vi "Microwave Amplifier Control Panel (No Objects).vi"(8 "error in (no error)":errorcluster) -> (0 "error out":errorcluster)   [LabVIEW 2012]
doc: "(Dynamic) A user-level application that simulates the physical front panel of the Instrument. Provide the user with buttons to manually control features of the instrument, and provide indicators of its current state."
uses:
  Microwave Amp/MicrowaveAmplifier.lvlib
panel:
  in  "VISA Resource Name":refnum<visa-resource-name>="GPIB0::12::INSTR"
  in  "Copy actual to set":bool
  in  "Populate fields with member data":bool
  in  "Read Remaining Time Delay":bool
  in  "Read Amplifier Status/Mode":bool
  in  "Standby":bool
  in  "stop":bool
  out "Mode":u16(ring) items=["SLEEP", "WARM-UP", "STANDBY", "OPERATE", "FAULT"]
  in  "Operate":bool
  in  "Read Reverse Power Out (W)":bool
  in  "Read Reverse Power Out (dBm)":bool
  in  "Read Forward Power Out (W)":bool
  in  "Read Forward Power out (dBm)":bool
  in  "Read Gain":bool
  in  "Set Gain":bool
  out "Remaining Heater Delay Time":dbl[unit]
  out "Reverse Power Out (dBm)":dbl
  out "Reverse Power Out (W)":dbl[unit]
  out "Forward Power Out (dBm)":dbl
  out "Forward Power Out (W)":dbl[unit]
  out "Gain (%)":dbl
  in  "GainSet":dbl
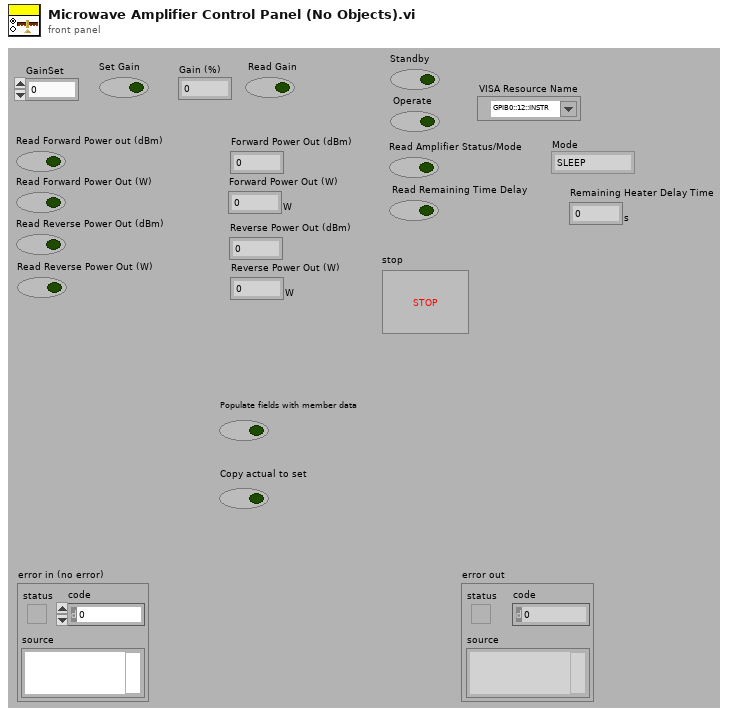
[diagram p1: front panel]
types:
  T1 = cluster{"Gain (%)":dbl, "Forward Power Out (dBm)":dbl, "Forward Power Out (W)":dbl[unit], "Reverse Power Out (dBm)":dbl, "Reverse Power Out (W)":dbl[unit], "Mode":u16, "Remaining Heater Delay Time (s)":dbl[unit]}
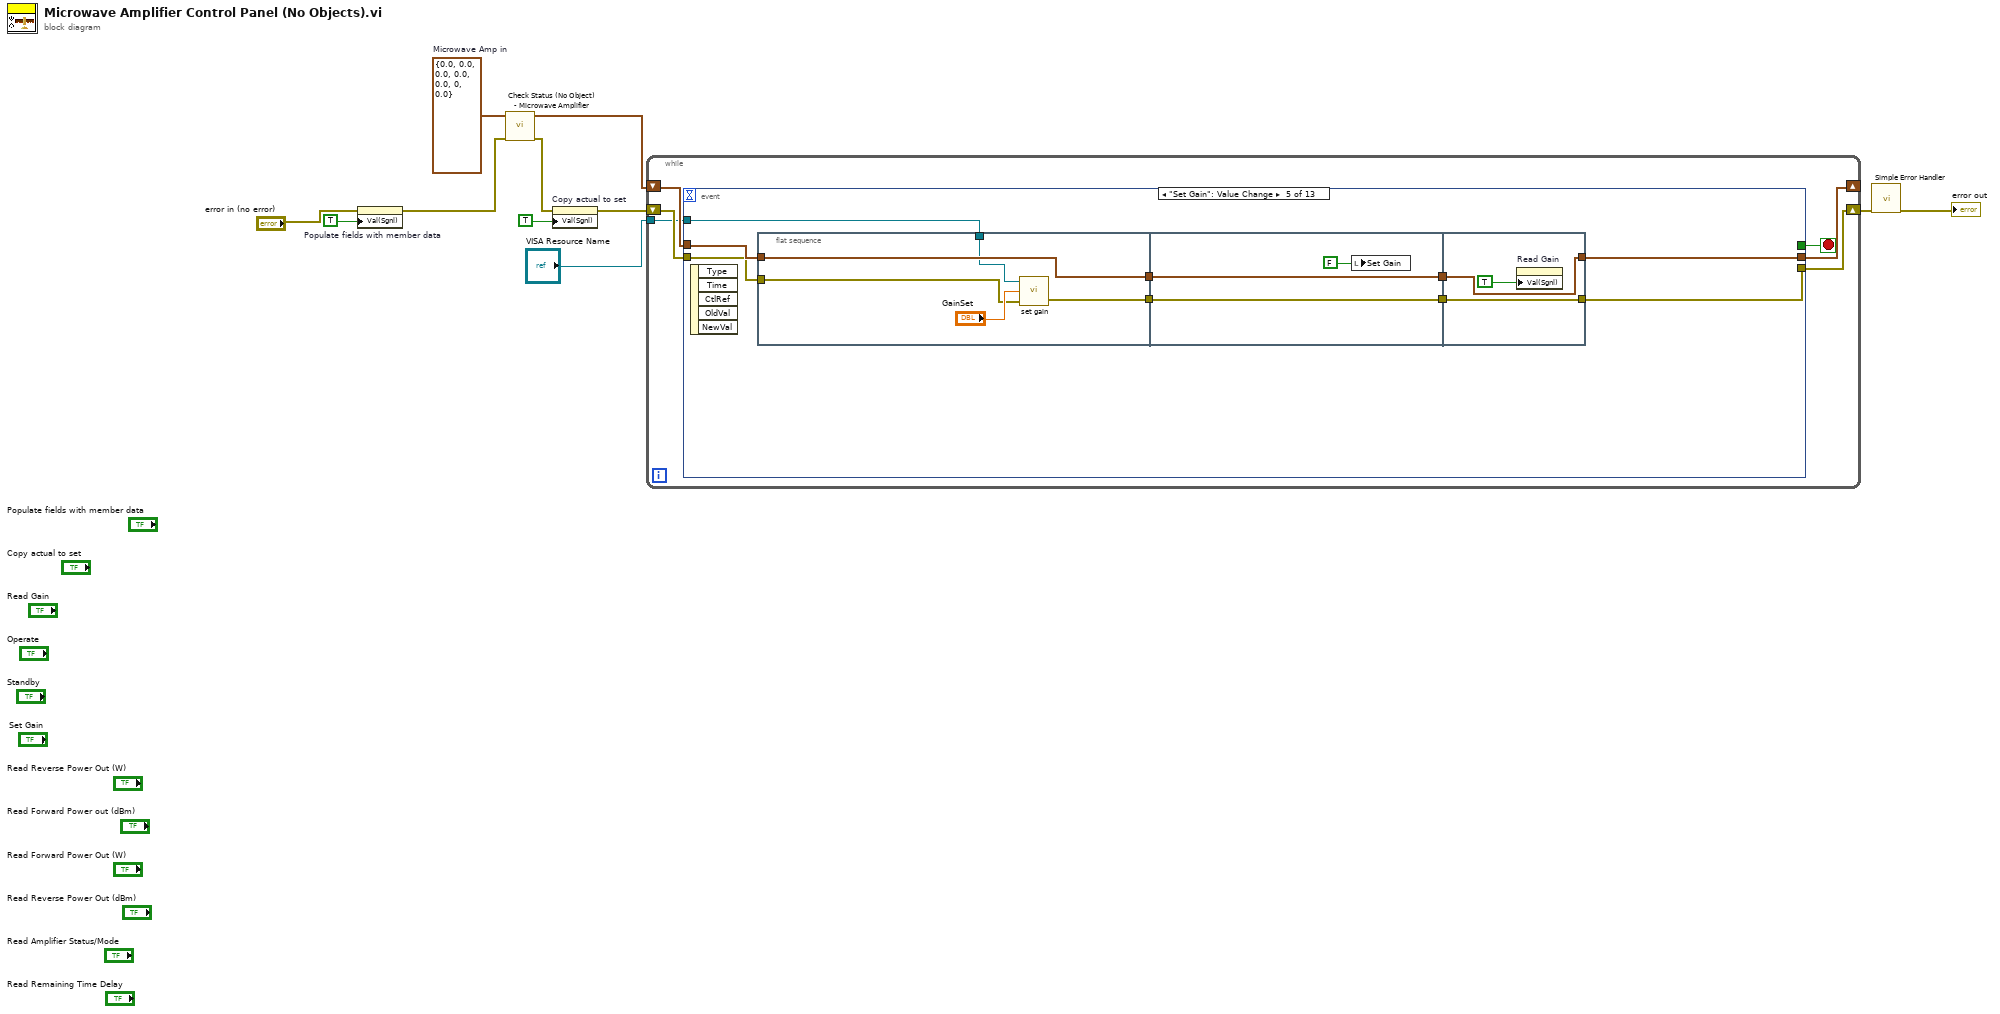
[diagram p0: block diagram]
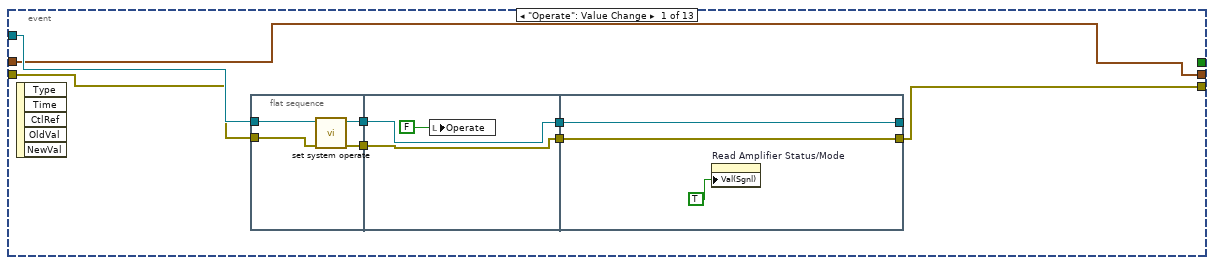
[diagram p2: hidden frame]
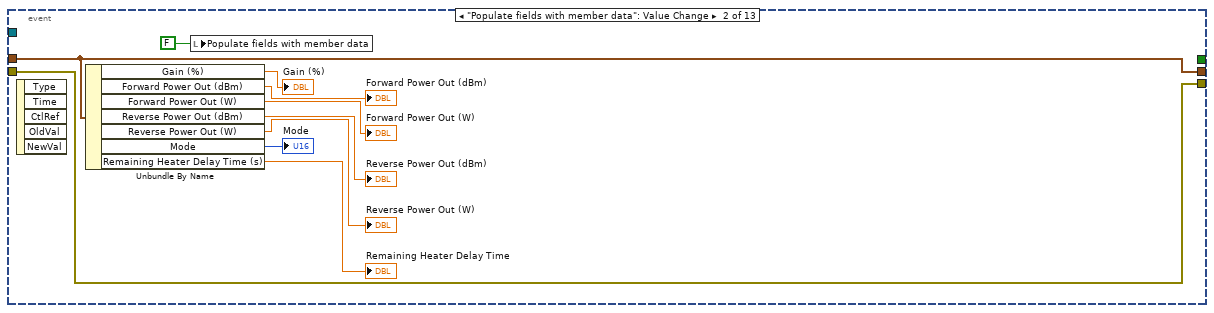
[diagram p3: hidden frame]
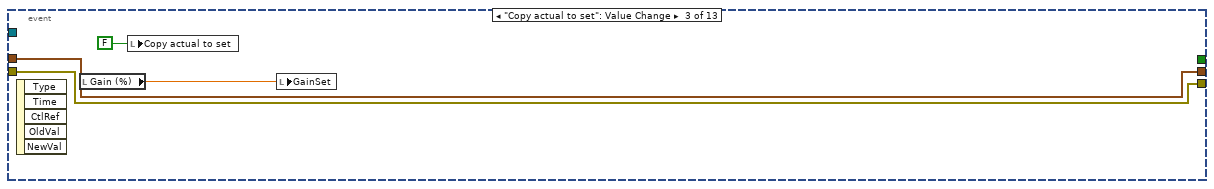
[diagram p4: hidden frame]
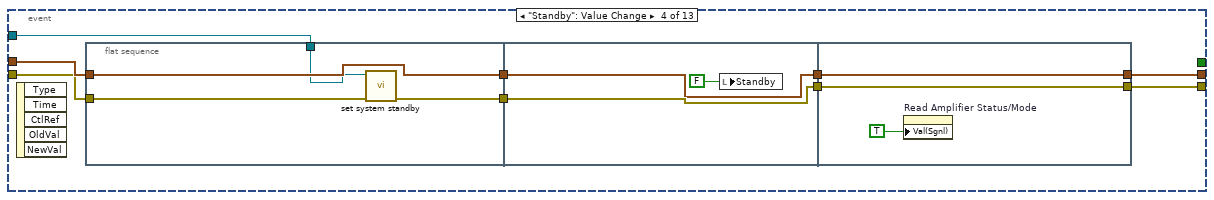
[diagram p5: hidden frame]
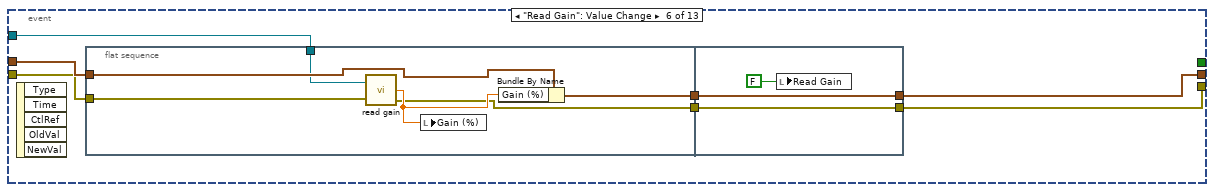
[diagram p6: hidden frame]
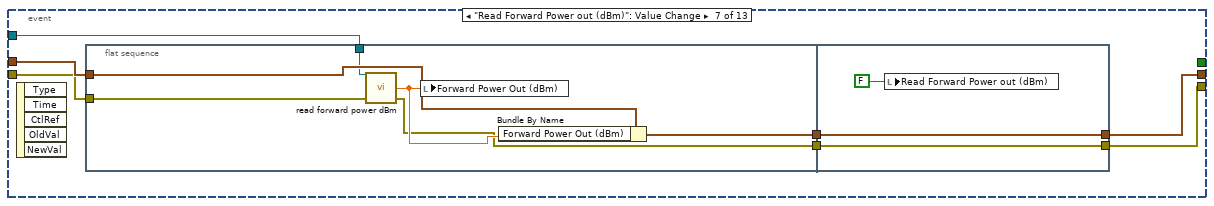
[diagram p7: hidden frame]
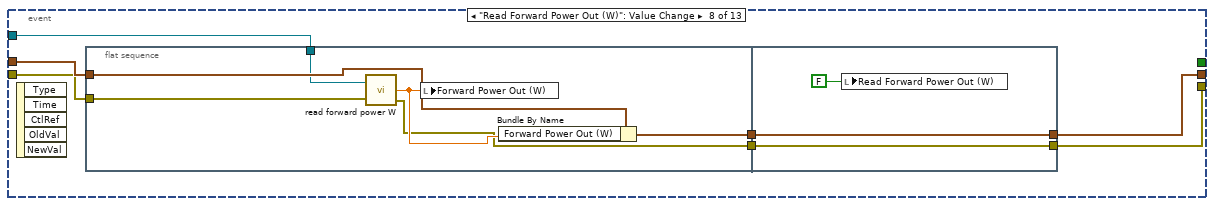
[diagram p8: hidden frame]
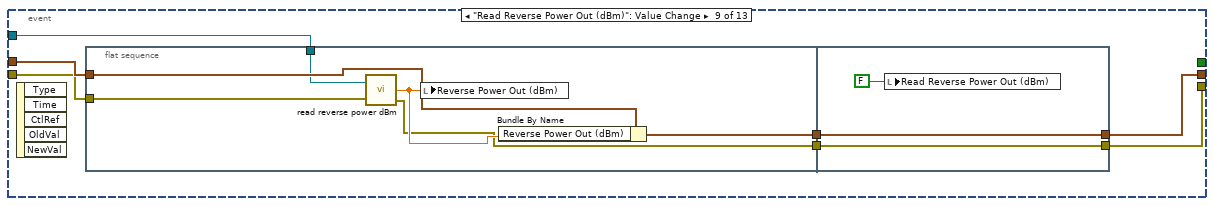
[diagram p9: hidden frame]
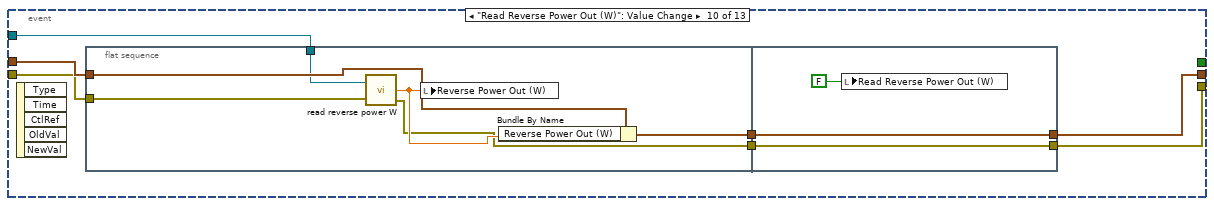
[diagram p10: hidden frame]
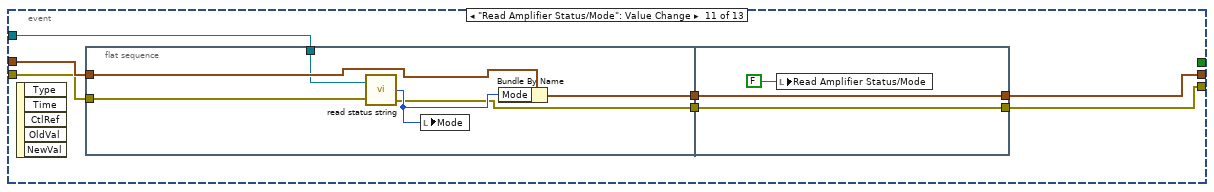
[diagram p11: hidden frame]
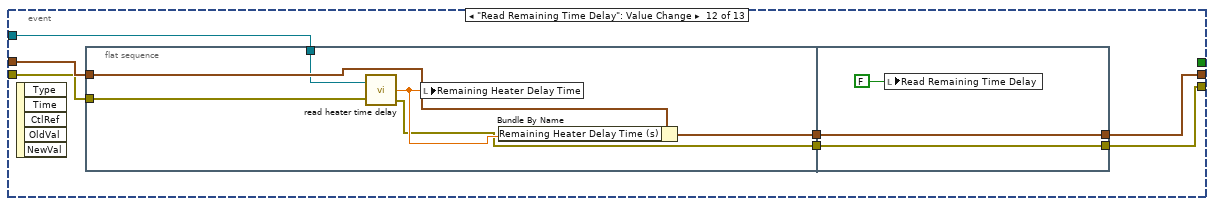
[diagram p12: hidden frame]
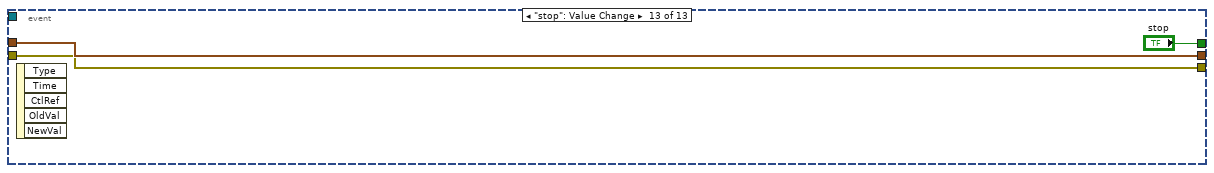
[diagram p13: hidden frame]
diagram:
  w5 = T1 {"Gain (%)"=0.0, "Forward Power Out (dBm)"=0.0, "Forward Power Out (W)"=0.0, "Reverse Power Out (dBm)"=0.0, "Reverse Power Out (W)"=0.0, "Mode"=0, "Remaining Heater Delay Time (s)"=0.0}  # Microwave Amp in
  n1 = property on="Populate fields with member data" class="Bool (strict)"(error in="error in (no error)", "Val(Sgnl)"=TRUE ("Value (Signaling)")) -> (error out=w3:errorcluster)  [unwired: 1 in, 1 out]
  n2 = call "Check Status (No Object) - Microwave Amplifier.vi"("error in (no error)"=w3, "Cluster In"=w5) -> ("error out"=w2:errorcluster, "Cluster Out"=w4:T1)  [unwired: 6 in, 2 out]
  n3 = property on="Copy actual to set" class="Bool (strict)"(error in=w2, "Val(Sgnl)"=TRUE ("Value (Signaling)")) -> (error out=w8:errorcluster)  [unwired: 1 in, 1 out]
  n4 = while {
    shift-right: [w17] -> w11
    shift-left: w8 -> [w14]
    shift-right: [w15] -> _
    shift-left: w4 -> [w13]
    tunnel: "VISA Resource Name" -> [w12]
    stop <- w16 stop-if-true
    n5 = event shown="[4] \"Set Gain\": Value Change" {
      selector: _ -> [_ _ _ _ _ _ _ _ _ _ _ _ _]
      dyn-events: _ -> [_ _ _ _ _ _ _ _ _ _ _ _ _]
      timeout: _ -> [_ _ _ _ _ _ _ _ _ _ _ _ _]
      tunnel: w14 -> [w20 w45 w48 w53 w74 w93 w107 w123 w139 w155 w171 w189 w201]
      tunnel: [w18 w45 w48 w57 w70 w90 w106 w122 w138 w154 w170 w186 w201] -> w17
      tunnel: [_ _ _ _ _ _ _ _ _ _ _ _ "stop"] -> w16
      tunnel: w13 -> [w19 w44 w49 w54 w75 w94 w110 w126 w142 w158 w174 w190 w202]
      tunnel: [w19 w44 w49 w55 w73 w92 w109 w125 w141 w157 w173 w188 w202] -> w15
      tunnel: w12 -> [w21 _ _ w50 w69 w89 w105 w121 w137 w153 w169 w185 _]
      event "Operate": Value Change {
        n6 = event-data() -> ()  [unwired: 1 in, 5 out]
        n7 = flat-sequence {
          tunnel: [w29] -> w25
          tunnel: [w28] -> w24
          tunnel: w20 -> [w27]
          tunnel: w21 -> [w26]
          tunnel: w25 -> [w31]
          tunnel: w24 -> [w30]
          tunnel: [w31] -> w23
          tunnel: [w30] -> w22
          tunnel: [w34] -> w18
          tunnel: [w35] -> _
          tunnel: w23 -> [w35]
          tunnel: w22 -> [w34]
          frame #0 {
            n8 = call "set system operate.vi"("error in (no error)"=w27, "VISA resource name"=w26) -> ("error out"=w28:errorcluster, "VISA resource name out"=w29:refnum<visa-resource-name>)  [unwired: 8 in]
          }
          frame #1 {
            n9 = local write "Operate"(FALSE ("Operate")) -> ()
          }
          frame #2 {
            n10 = property on="Read Amplifier Status/Mode" class="Bool (strict)"("Val(Sgnl)"=TRUE ("Value (Signaling)")) -> ()  [unwired: 2 in, 2 out]
          }
        }
      }
      event "Populate fields with member data": Value Change {
        n11 = event-data() -> ()  [unwired: 1 in, 5 out]
        n12 = Unbundle By Name(w44) -> ("Gain (%)"=→"Gain (%)":dbl, "Forward Power Out (dBm)"=→"Forward Power Out (dBm)":dbl, "Forward Power Out (W)"=→"Forward Power Out (W)":dbl[unit], "Reverse Power Out (dBm)"=→"Reverse Power Out (dBm)":dbl, "Reverse Power Out (W)"=→"Reverse Power Out (W)":dbl[unit], "Mode"=→"Mode":u16, "Remaining Heater Delay Time (s)"=→"Remaining Heater Delay Time":dbl[unit])
        n13 = local write "Populate fields with member data"(FALSE ("Populate fields with member data")) -> ()
      }
      event "Copy actual to set": Value Change {
        n14 = event-data() -> ()  [unwired: 1 in, 5 out]
        n15 = local read "Gain (%)"() -> (w46:dbl)
        n16 = local write "Copy actual to set"(FALSE ("Copy actual to set")) -> ()
        n17 = local write "GainSet"(w46) -> ()
      }
      event "Standby": Value Change {
        n18 = event-data() -> ()  [unwired: 1 in, 5 out]
        n19 = flat-sequence {
          tunnel: [w62] -> w58
          tunnel: [w61] -> w56
          tunnel: w54 -> [w61]
          tunnel: w53 -> [w60]
          tunnel: w50 -> [w59]
          tunnel: w58 -> [w64]
          tunnel: w56 -> [w63]
          tunnel: [w64] -> w52
          tunnel: [w63] -> w51
          tunnel: [w67] -> w55
          tunnel: [w68] -> w57
          tunnel: w52 -> [w68]
          tunnel: w51 -> [w67]
          frame #0 {
            n20 = call "set system standby.vi"("error in (no error)"=w60, "VISA resource name"=w59) -> ("error out"=w62:errorcluster)  [unwired: 8 in, 1 out]
          }
          frame #1 {
            n21 = local write "Standby"(FALSE ("Operate")) -> ()
          }
          frame #2 {
            n22 = property on="Read Amplifier Status/Mode" class="Bool (strict)"("Val(Sgnl)"=TRUE ("Value (Signaling)")) -> ()  [unwired: 2 in, 2 out]
          }
        }
      }
      event "Set Gain": Value Change {
        n23 = event-data() -> ()  [unwired: 1 in, 5 out]
        n24 = flat-sequence {
          tunnel: [w81] -> w77
          tunnel: w75 -> [w80]
          tunnel: w74 -> [w79]
          tunnel: [w80] -> w71
          tunnel: w69 -> [w78]
          tunnel: w77 -> [w84]
          tunnel: [w84] -> w76
          tunnel: [w83] -> w72
          tunnel: w71 -> [w83]
          tunnel: [w88] -> w70
          tunnel: w76 -> [w88]
          tunnel: [w86] -> w73
          tunnel: w72 -> [w86]
          frame #0 {
            n25 = call "set gain.vi"("error in (no error)"=w79, "Gain"="GainSet", "VISA resource name"=w78) -> ("error out"=w81:errorcluster)  [unwired: 1 out]
          }
          frame #1 {
            n26 = local write "Set Gain"(FALSE ("Set Gain")) -> ()
          }
          frame #2 {
            n27 = property on="Read Gain" class="Bool (strict)"("Val(Sgnl)"=TRUE ("Value (Signaling)")) -> ()  [unwired: 2 in, 2 out]
          }
        }
      }
      event "Read Gain": Value Change {
        n28 = event-data() -> ()  [unwired: 1 in, 5 out]
        n29 = flat-sequence {
          tunnel: [w99] -> w95
          tunnel: w94 -> [w97]
          tunnel: w93 -> [w98]
          tunnel: [w100] -> w91
          tunnel: w89 -> [w96]
          tunnel: [w103] -> w90
          tunnel: w95 -> [w103]
          tunnel: [w102] -> w92
          tunnel: w91 -> [w102]
          frame #0 {
            n30 = call "read gain.vi"("VISA resource name"=w96, "error in (no error)"=w98) -> ("Gain (%)"=w101:dbl, "error out"=w99:errorcluster)  [unwired: 1 out]
            n31 = local write "Gain (%)"(w101) -> ()
            n32 = Bundle By Name(cluster=w97, "Gain (%)"=w101) -> (w100:T1)
          }
          frame #1 {
            n33 = local write "Read Gain"(FALSE ("Read Gain")) -> ()
          }
        }
      }
      event "Read Forward Power out (dBm)": Value Change {
        n34 = event-data() -> ()  [unwired: 1 in, 5 out]
        n35 = flat-sequence {
          tunnel: [w113] -> w111
          tunnel: w110 -> [w114]
          tunnel: [w116] -> w108
          tunnel: w107 -> [w115]
          tunnel: w105 -> [w112]
          tunnel: [w120] -> w106
          tunnel: w111 -> [w120]
          tunnel: [w118] -> w109
          tunnel: w108 -> [w118]
          frame #0 {
            n36 = call "read forward power dBm.vi"("error in (no error)"=w115, "VISA resource name"=w112) -> ("error out"=w113:errorcluster, "forward power (dBm)"=w117:dbl)  [unwired: 1 in, 1 out]
            n37 = local write "Forward Power Out (dBm)"(w117) -> ()
            n38 = Bundle By Name(cluster=w114, "Forward Power Out (dBm)"=w117) -> (w116:T1)
          }
          frame #1 {
            n39 = local write "Read Forward Power out (dBm)"(FALSE ("Read Forward Power out (dBm)")) -> ()
          }
        }
      }
      event "Read Forward Power Out (W)": Value Change {
        n40 = event-data() -> ()  [unwired: 1 in, 5 out]
        n41 = flat-sequence {
          tunnel: [w131] -> w127
          tunnel: w126 -> [w129]
          tunnel: [w132] -> w124
          tunnel: w123 -> [w130]
          tunnel: w121 -> [w128]
          tunnel: [w136] -> w122
          tunnel: w127 -> [w136]
          tunnel: [w134] -> w125
          tunnel: w124 -> [w134]
          frame #0 {
            n42 = call "read forward power W.vi"("VISA resource name"=w128, "error in (no error)"=w130) -> ("foward power (W)"=w133:dbl[unit], "error out"=w131:errorcluster)  [unwired: 1 out]
            n43 = local write "Forward Power Out (W)"(w133) -> ()
            n44 = Bundle By Name(cluster=w129, "Forward Power Out (W)"=w133) -> (w132:T1)
          }
          frame #1 {
            n45 = local write "Read Forward Power Out (W)"(FALSE ("Read Forward Power Out (W)")) -> ()
          }
        }
      }
      event "Read Reverse Power Out (dBm)": Value Change {
        n46 = event-data() -> ()  [unwired: 1 in, 5 out]
        n47 = flat-sequence {
          tunnel: [w147] -> w143
          tunnel: w142 -> [w145]
          tunnel: [w148] -> w140
          tunnel: w139 -> [w146]
          tunnel: w137 -> [w144]
          tunnel: [w151] -> w138
          tunnel: w143 -> [w151]
          tunnel: [w150] -> w141
          tunnel: w140 -> [w150]
          frame #0 {
            n48 = call "read reverse power dBm.vi"("VISA resource name"=w144, "error in (no error)"=w146) -> ("reverse power (dBm)"=w149:dbl, "error out"=w147:errorcluster)  [unwired: 1 out]
            n49 = local write "Reverse Power Out (dBm)"(w149) -> ()
            n50 = Bundle By Name(cluster=w145, "Reverse Power Out (dBm)"=w149) -> (w148:T1)
          }
          frame #1 {
            n51 = local write "Read Reverse Power Out (dBm)"(FALSE ("Read Reverse Power Out (dBm)")) -> ()
          }
        }
      }
      event "Read Reverse Power Out (W)": Value Change {
        n52 = event-data() -> ()  [unwired: 1 in, 5 out]
        n53 = flat-sequence {
          tunnel: [w162] -> w159
          tunnel: w158 -> [w161]
          tunnel: [w165] -> w156
          tunnel: w155 -> [w163]
          tunnel: w153 -> [w160]
          tunnel: [w167] -> w154
          tunnel: w159 -> [w167]
          tunnel: [w166] -> w157
          tunnel: w156 -> [w166]
          frame #0 {
            n54 = call "read reverse power W.vi"("VISA resource name"=w160, "error in (no error)"=w163) -> ("Reverse Power (W)"=w164:dbl[unit], "error out"=w162:errorcluster)  [unwired: 1 out]
            n55 = local write "Reverse Power Out (W)"(w164) -> ()
            n56 = Bundle By Name(cluster=w161, "Reverse Power Out (W)"=w164) -> (w165:T1)
          }
          frame #1 {
            n57 = local write "Read Reverse Power Out (W)"(FALSE ("Read Reverse Power Out (W)")) -> ()
          }
        }
      }
      event "Read Amplifier Status/Mode": Value Change {
        n58 = event-data() -> ()  [unwired: 1 in, 5 out]
        n59 = flat-sequence {
          tunnel: [w178] -> w175
          tunnel: w174 -> [w177]
          tunnel: [w181] -> w172
          tunnel: w171 -> [w179]
          tunnel: w169 -> [w176]
          tunnel: [w184] -> w170
          tunnel: w175 -> [w184]
          tunnel: [w182] -> w173
          tunnel: w172 -> [w182]
          frame #0 {
            n60 = call "read status string.vi"("VISA resource name"=w176, "error in (no error)"=w179) -> ("Mode"=w180:u16, "error out"=w178:errorcluster)  [unwired: 1 out]
            n61 = local write "Mode"(w180) -> ()
            n62 = Bundle By Name(cluster=w177, "Mode"=w180) -> (w181:T1)
          }
          frame #1 {
            n63 = local write "Read Amplifier Status/Mode"(FALSE ("Read Amplifier Status")) -> ()
          }
        }
      }
      event "Read Remaining Time Delay": Value Change {
        n64 = event-data() -> ()  [unwired: 1 in, 5 out]
        n65 = flat-sequence {
          tunnel: [w195] -> w191
          tunnel: w190 -> [w194]
          tunnel: w189 -> [w193]
          tunnel: [w196] -> w187
          tunnel: w185 -> [w192]
          tunnel: [w200] -> w186
          tunnel: w191 -> [w200]
          tunnel: [w198] -> w188
          tunnel: w187 -> [w198]
          frame #0 {
            n66 = call "read heater time delay.vi"("VISA resource name"=w192, "error in (no error)"=w193) -> ("Heater delay time (s)"=w197:dbl[unit], "error out"=w195:errorcluster)  [unwired: 1 out]
            n67 = local write "Remaining Heater Delay Time"(w197) -> ()
            n68 = Bundle By Name(cluster=w194, "Remaining Heater Delay Time (s)"=w197) -> (w196:T1)
          }
          frame #1 {
            n69 = local write "Read Remaining Time Delay"(FALSE ("Read Remaining Time Delay")) -> ()
          }
        }
      }
      event "stop": Value Change {
        n70 = event-data() -> ()  [unwired: 1 in, 5 out]
      }
    }
  }
  n71 = call <vilib>:"Simple Error Handler.vi"("error in (no error)"=w11) -> ("error out"=→"error out":errorcluster)  [unwired: 1 in, 7 out]
